vi "Library - Friends.vi"(7 "Msg Chain":string, 8 "error in (no error)":errorcluster {"code" format="Error %.0f"}, 10 "Libraries":refnum<class "Library Documentation.lvclass">[](array[class]), 11 "VIDoc Printer - Confluence In":refnum<class "VIDoc Printer - Confluence.lvclass">) -> (0 "error out":errorcluster {"code" format="Error %.0f"}, 3 "VIDoc Printer - Confluence Out":refnum<class "VIDoc Printer - Confluence.lvclass">)   [LabVIEW 2023, in "VIDoc Printer - Confluence.lvlib" / "VIDoc Printer - Confluence.lvclass"]
uses:
  VIDoc Printer - Confluence.lvclass
  C:/projects/DMC/Tooling/Git-Action-Service/Source/Documentation Generation/Printers/Printer/VIDoc Printer.lvclass
  Parsing/Library Documentation/Library Documentation.lvclass
  Parsing/Library Documentation/Library Documentation.lvclass/Library Documentation.ctl
  Confluence Formatting/Types/Format Combo Box.ctl
  VIDoc Printer - Confluence.lvclass/VIDoc Printer - Confluence.ctl
  Accessors/Get Library Inheritance Expand.vi
  Parsing/Library Documentation/Get Library Info.vi
  Parsing/Library Documentation/Get Name.vi
  Printer/VIDoc Printer.lvclass
  UI Interaction/UI Interaction.lvclass
  Confluence Formatting/Confluence Formatting.lvlib
  C:/projects/DMC/Tooling/Git-Action-Service/Source/Documentation Generation/Printers/Confluence Printer/VIDoc Printer - Confluence.lvclass
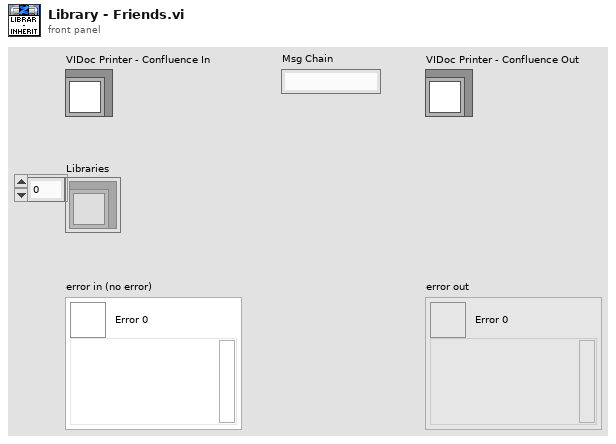
[diagram p1: front panel]
types:
  T1 = typedef "Confluence Formatting.lvlib/Format Combo Box.ctl" = string
  T2 = typedef "VIDoc Parsing.lvlib/Base Library Info Cluster.ctl" = cluster{"Name":string, "Icon":T3, "Version":cluster{"Major":u16, "Minor":u16, "Fix":u16, "Build":u16}, "Description":string, "Path":path, "Friends":string[], "Library Scope":enum32{"invalid scope", "public", "private", "protected", "community"}, "Qualified Name":string}
  T3 = typedef "imagedata.ctl" = cluster{"image type":i32, "image depth":i32, "image":u8[], "mask":u8[], "colors":u32[], "Rectangle":cluster{"left":i16, "top":i16, "right":i16, "bottom":i16}}
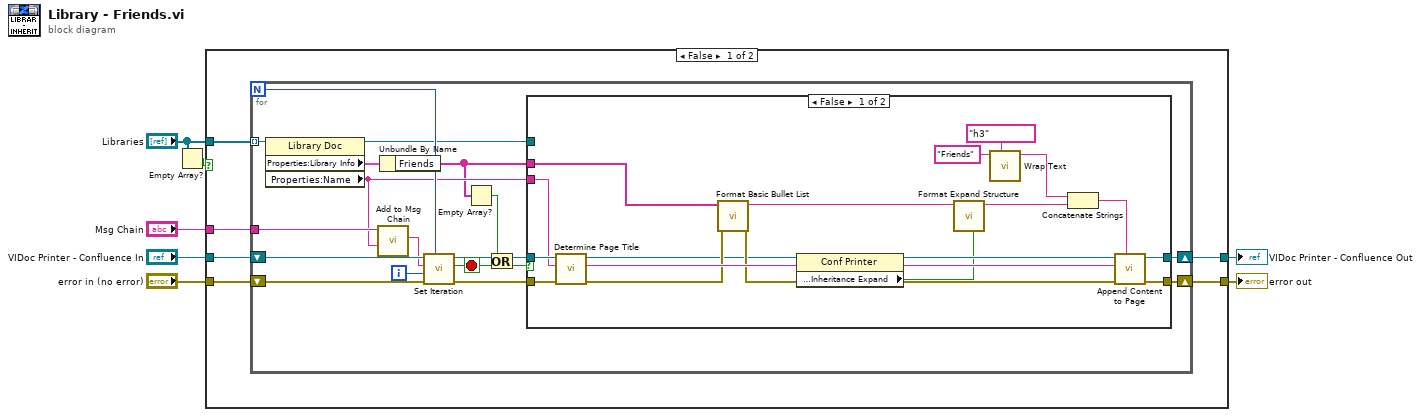
[diagram p0: block diagram]
diagram:
  n1 = Empty Array?(array="Libraries") -> (empty?=w7:bool)
  n2 = case shown="False" w7 {
    tunnel: [w13 w52] -> w6
    tunnel: [w12 w53] -> w5
    tunnel: "error in (no error)" -> [w11 w52]
    tunnel: "Libraries" -> [w10 _]
    tunnel: "VIDoc Printer - Confluence In" -> [w9 w53]
    tunnel: "Msg Chain" -> [w8 _]
    frame False {
      n3 = for {
        N -> [w24]
        shift-right: [w29] -> w13
        shift-left: w11 -> [w27]
        shift-right: [w30] -> w12
        shift-left: w9 -> [w28]
        tunnel: w10 -> [w31] mode=indexing
        tunnel: w8 -> [w22]
        i -> [w23]
        stop <- w19 stop-if-true
        n4 = property class="Library Doc"(reference=w31) -> (reference out=w18:refnum<class "Library Documentation.lvclass">, "Properties:Library Info"=w17:T2, "Properties:Name"=w21:string)  [unwired: 1 in, 1 out]
        n5 = call "Add to Msg Chain.vi"("New"=w21, "Msg Chain in"=w22) -> ("Msg Chain out"=w20:string)  [unwired: 9 in]
        n6 = Unbundle By Name(w17) -> ("Friends"=w16:string[])
        n7 = call "Set Iteration.vi"("Progress Max"=w24, "error in (no error)"=w27, "Progress Value"=w23, "Message (No Message Update)"=w20, "VIDoc Printer In"=w28) -> ("error out"=w25:errorcluster, "Abort?"=w19:bool, "VIDoc Printer Out"=w26:refnum<class "VIDoc Printer - Confluence.lvclass">)  [unwired: 4 in]
        n8 = Empty Array?(array=w16) -> (empty?=w14:bool)
        n9 = Or(x=w14, y=w19) -> (x .or. y?=w15:bool)
        n10 = case shown="False" w15 {
          tunnel: [w48 w50] -> w30
          tunnel: [w47 w51] -> w29
          tunnel: w26 -> [w45 w50]
          tunnel: w25 -> [w44 w51]
          tunnel: w21 -> [w43 _]
          tunnel: w18 -> [_ _]
          tunnel: w16 -> [w35 _]
          frame False {
            n11 = call "Determine Page Title.vi"("error in (no error)"=w44, "Name"=w43, "VIDoc Printer - Confluence In"=w45) -> ("error out"=w39:errorcluster, "Page Title"=w49:string, "VIDoc Printer - Confluence Out"=w37:refnum<class "VIDoc Printer - Confluence.lvclass">)  [unwired: 5 in, 1 out]
            n12 = call "Format Basic Bullet List.vi"("Error in"=w39, "String Array"=w35) -> ("Error out"=w38:errorcluster, "Bullet List"=w36:string)  [unwired: 8 in]
            n13 = property class="Conf Printer"(reference=w37) -> (reference out=w34:refnum<class "VIDoc Printer - Confluence.lvclass">, "Properties:Expand?:Library:Inheritance Expand"=w32:bool)  [unwired: 1 in, 1 out]
            n14 = call "Format Expand Structure.vi"("Enable? (T)"=w32, "Content"=w36) -> ("Expand String"=w33:string)  [unwired: 8 in, 1 out]
            n15 = call "Wrap Text.vi"("Formatting"=T1 "h3", "String"="Friends") -> ("Wrapped String"=w41:string)  [unwired: 8 in, 1 out]
            n16 = Concatenate Strings(w41, w33) -> (w40:string)
            n17 = call "Append Content to Page.vi"("Page Content"=w40, "error in (no error)"=w38, "Page Title"=w49, "VIDoc Printer - Confluence In"=w34) -> ("error out"=w47:errorcluster, "VIDoc Printer - Confluence Out"=w48:refnum<class "VIDoc Printer - Confluence.lvclass">)  [unwired: 6 in]
          }
          frame True {
          }
        }
      }
    }
    frame True {
    }
  }
  "error out" <- w6
  "VIDoc Printer - Confluence Out" <- w5
